vi "Clean up Wire on Inner Terminal.vi"(8 "error in (no error)":errorcluster, 11 "InnerTerminal in":refnum<vi>) -> (0 "error out":errorcluster, 3 "InnerTerminal out":refnum<vi>)   [LabVIEW 2020, in "JKI State Machine API.lvlib" / "JKI SM.lvclass"]
uses:
  JKI SM/JKI SM.lvclass
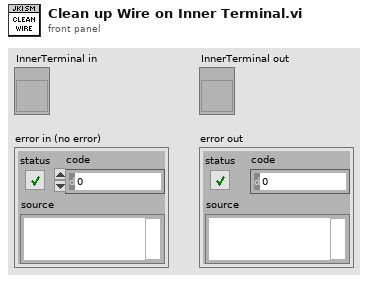
[diagram p1: front panel]
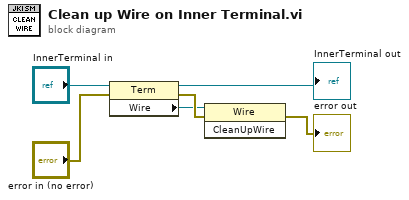
[diagram p0: block diagram]
diagram:
  n1 = property class="Term"(reference="InnerTerminal in", error in="error in (no error)") -> (reference out=→"InnerTerminal out":refnum<vi>, error out=w3:errorcluster, "Wire"=w2:refnum<vi>)
  n2 = invoke class="Wire" method="CleanUpWire"(reference=w2, error in=w3) -> (error out=→"error out":errorcluster)  [unwired: 1 in, 2 out]
